vi "FTW-Actor-LocalMessage-RegisterForShutdown.vi"(0 "FTW-ActorInstance In":refnum<class "FTW-ActorInstance.lvclass">, 11 "error in":errorcluster) -> (4 "FTW-ActorInstance Out":refnum<class "FTW-ActorInstance.lvclass">, 8 "ShutdownEventRegistrationRefnum":refnum<event-registration>, 15 "error out":errorcluster)   [LabVIEW 2015, in "FTW-ActorInstance.lvclass"]
doc: "Use this VI to register for the actor shutdown event for creating async workers"
uses:
  FTW-ActorInstance.lvclass
  FTW-ActorInstance.lvclass/FTW-ActorInstance.ctl
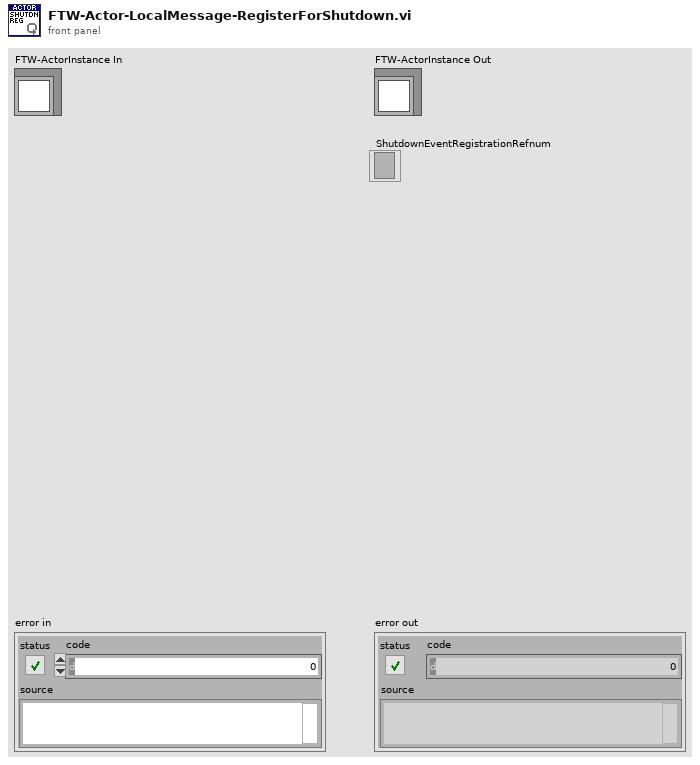
[diagram p1: front panel]
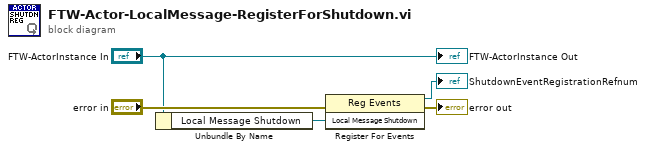
[diagram p0: block diagram]
diagram:
  n1 = Unbundle By Name("FTW-ActorInstance In") -> ("Local Message Shutdown"=w4:refnum<user-event>)
  n2 = register-events(error in="error in", w4) -> (reference out=→"ShutdownEventRegistrationRefnum":refnum<event-registration>, error out=→"error out":errorcluster)  [unwired: 1 in]
  "FTW-ActorInstance Out" <- "FTW-ActorInstance In"
